vi "Scan Setup.vi"(8 "error in (no error)":errorcluster, 11 "Magnetic Field Lakeshore Scan in":refnum<class "Magnetic Field Lakeshore Scan.lvclass">) -> (0 "error out":errorcluster, 3 "Magnetic Field Lakeshore Scan out":refnum<class "Magnetic Field Lakeshore Scan.lvclass">)   [LabVIEW 2023, in "Magnetic Field Lakeshore Scan.lvclass"]
doc: "Configure the Instrument based on the class member fields. This step comes after the user has closed the \"Scan Setup\" window and before the actual scan -- so instruments are configured with the user's specified settings."
uses:
  Magnetic Field Lakeshore Scan.lvclass
  Magnetic Field Lakeshore Scan.lvclass/Magnetic Field Lakeshore Scan.ctl
  Scanner/Scanner.lvclass
  Instruments/Utility Classes/Scannable/Scannable.lvclass
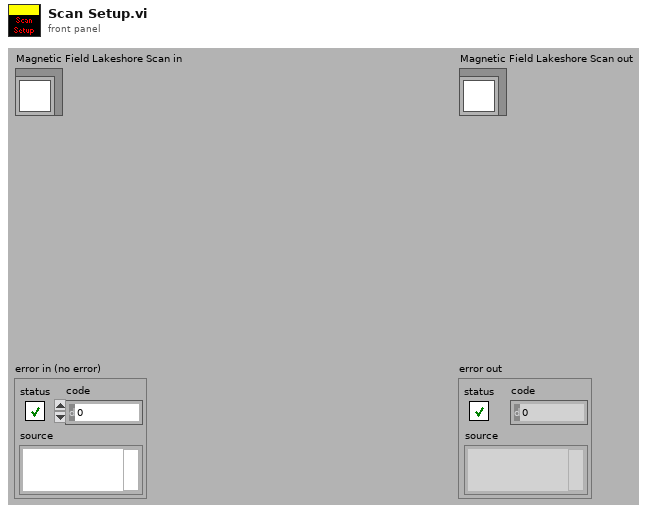
[diagram p1: front panel]
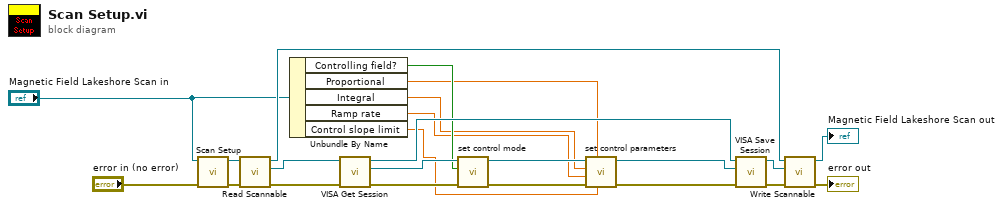
[diagram p0: block diagram]
diagram:
  n1 = call-parent "Scan Setup.vi"("error in (no error)"="error in (no error)", "Scanner in"="Magnetic Field Lakeshore Scan in") -> ("error out"=w16:errorcluster, "Scanner out"=w20:refnum<class "Magnetic Field Lakeshore Scan.lvclass">)  [unwired: 8 in]
  n2 = call-dynamic "Read Scannable.vi"("error in (no error)"=w16, "Scanner.lvclass in"=w20) -> ("error out"=w15:errorcluster, "Scannable.lvclass"=w18:refnum<class "Scannable.lvclass">, "Scanner.lvclass out"=w19:refnum<class "Magnetic Field Lakeshore Scan.lvclass">)  [unwired: 7 out]
  n3 = Unbundle By Name("Magnetic Field Lakeshore Scan in") -> ("Controlling field?"=w5:bool, "Proportional"=w4:dbl, "Integral"=w3:dbl[unit], "Ramp rate"=w2:dbl[unit], "Control slope limit"=w1:dbl[unit])
  n4 = call-dynamic "VISA Get Session.vi"("error in (no error)"=w15, "Instrument.lvclass in"=w18) -> ("error out"=w7:errorcluster, "VISA Resource Name"=w9:refnum<visa-resource-name>, "Instrument.lvclass out"=w11:refnum<class "Scannable.lvclass">)  [unwired: 7 out]
  n5 = call "set control mode.vi"("error in (no error)"=w7, "Start/stop controlling field"=w5, "VISA session"=w9) -> ("error out"=w6:errorcluster, "dup VISA session"=w8:refnum<visa-resource-name>)  [unwired: 7 in]
  n6 = call "set control parameters.vi"("Control slope limit (10 V/min)"=w1, "Proportional (10)"=w4, "error in (no error)"=w6, "Ramp rate (3500 Gs/min)"=w2, "Integral (1 s)"=w3, "VISA session"=w8) -> ("error out"=w14:errorcluster, "dup VISA session"=w17:refnum<visa-resource-name>)  [unwired: 4 in]
  n7 = call-dynamic "VISA Save Session.vi"("error in (no error)"=w14, "VISA Resource Name"=w17, "Instrument.lvclass in"=w11) -> ("error out"=w13:errorcluster, "Instrument.lvclass out"=w10:refnum<class "Scannable.lvclass">)  [unwired: 7 out]
  n8 = call-dynamic "Write Scannable.vi"("error in (no error)"=w13, "Scannable.lvclass"=w10, "Scanner.lvclass in"=w19) -> ("error out"=→"error out":errorcluster, "Scanner.lvclass out"=→"Magnetic Field Lakeshore Scan out":refnum<class "Magnetic Field Lakeshore Scan.lvclass">)  [unwired: 7 out]
